vi "Build Installer with API.vi"(8 "error in (no error)":errorcluster, 11 "PostBuildSupport in":refnum<class "PostBuildSupport.lvclass">) -> (0 "error out":errorcluster, 3 "PostBuildSupport out":refnum<class "PostBuildSupport.lvclass">)   [LabVIEW 2019, in "PostBuildSupport.lvclass"]
uses:
  PostBuildSupport.lvclass
  PostBuildSupport.lvclass/PostBuildSupport.ctl
  <vilib>/AppBuilder/IB_Classes/Destination/IB_Destination.lvclass
  <vilib>/AppBuilder/IB_Classes/Source/IB_Source.lvclass
  <vilib>/AppBuilder/IB_Classes/Dest_NI_NIPath/Dest_NI_NIPath.lvclass
  <vilib>/AppBuilder/AB_API/EXE/NI_AB_API_EXE.lvclass
  <vilib>/AppBuilder/IB_Classes/Installer/Installer.lvclass
panel:
  in  "Cancel Button":bool
  out "Progress Bar":u8(slide) caption="The build is complete. You can locate the build at\nC:\\user\\patrick\\git\\PPMS-Monitor-and-Control\\builds\\PPMS Monitor and Control\\Application." scale=0.0..100.0
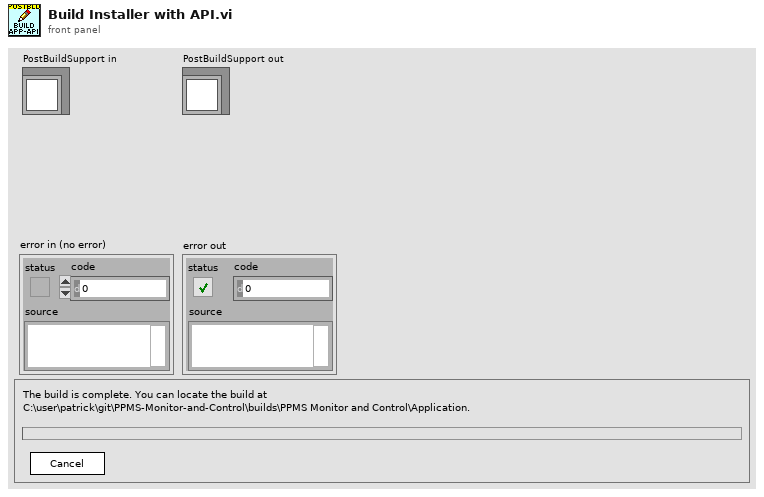
[diagram p1: front panel]
types:
  T1 = enum8{"Enabled", "Disabled", "Disabled and Grayed Out"}
  T2 = typedef "IB_Installer.ctl" = cluster{"Destination":refnum<class "IB_Destination.lvclass">[], "Source":refnum<class "IB_Source.lvclass">[], "buildObject":T3, "defaultDir":string, "platform":string, "author":string, "productName":string, "buildSpecName":string, "hide":bool, "requireLVDevSys":bool, "autoIncrement":bool, "includeError":bool, "readmeID":string, "buildLocation":path, "readmePath":path, "mediaSize":u16, "language":T4, "productVersion":T5, "preview":bool, "programmatic":bool, "progressBarEvents":T6, "userLog_Path":path, "shortcutAddresses":T8[], "EXE_Install Address":string, "EXE_Uninstall Address":string, "additional NIPaths":refnum<class "Dest_NI_NIPath.lvclass">[], "web service itemIDs":string[], "installerName":string}
  T3 = typedef "ItemRef.ctl" = u64
  T4 = typedef "CDK_sTypeDef_Languages.ctl" = u16
  T5 = typedef "CDK_sTypeDef_ProductVersion.ctl" = cluster{"Major":u8, "Minor":u8, "Update":u16}
  T6 = typedef "provcom_ProgressBar_Events.ctl" = cluster{"newJob":refnum<user-event>, "newItem":refnum<user-event>, "errorMsg":T7, "cancel":refnum<user-event>}
  T7 = typedef "mxLvBuildError.ctl" = refnum<user-event>
  T8 = typedef "CDK_sTypeDef_ShortcutAddress.ctl" = cluster{"file":string, "shortcut":string}
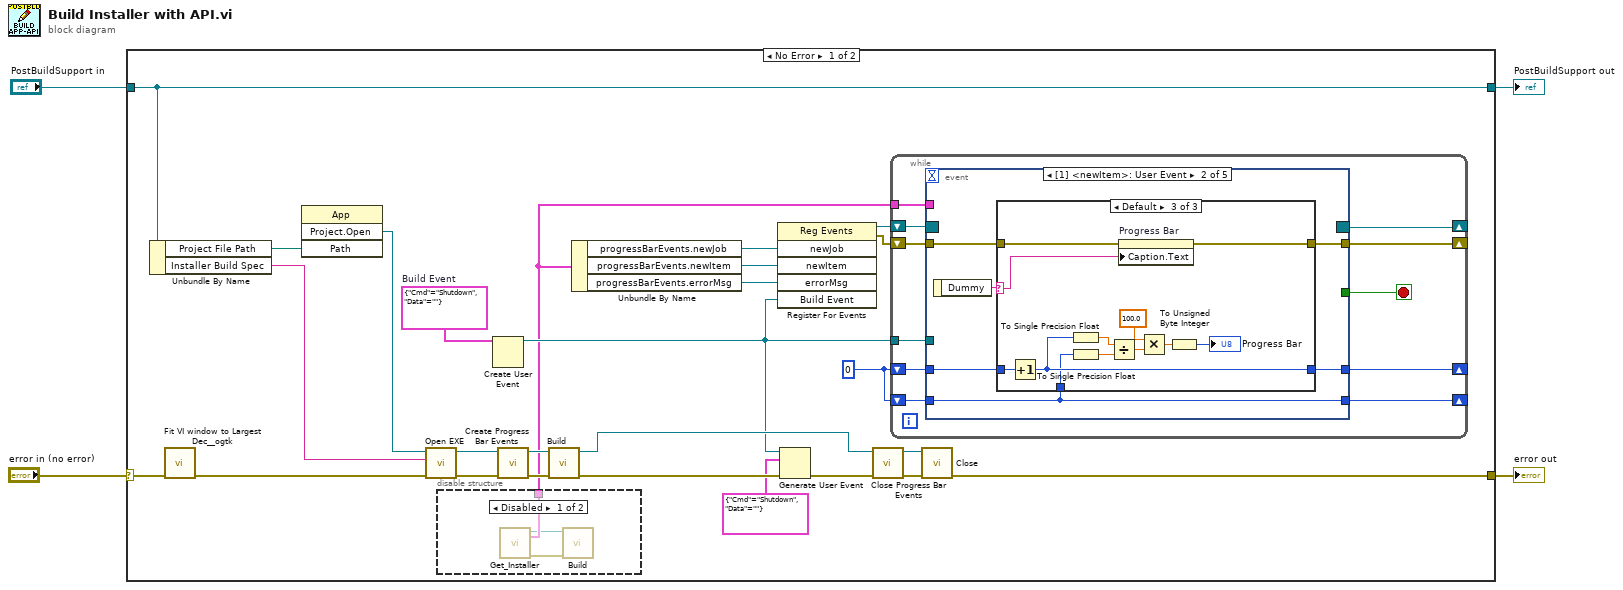
[diagram p0: block diagram]
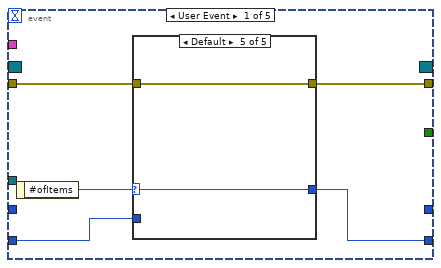
[diagram p3: hidden frame]
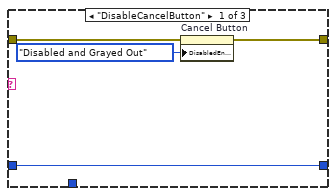
[diagram p8: hidden frame]
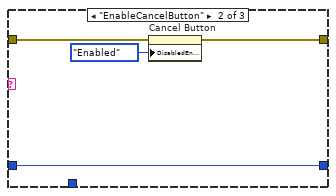
[diagram p9: hidden frame]
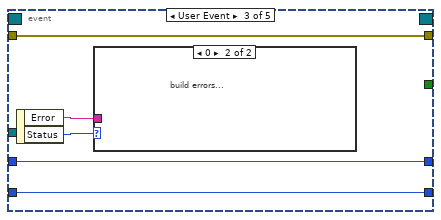
[diagram p10: hidden frame]
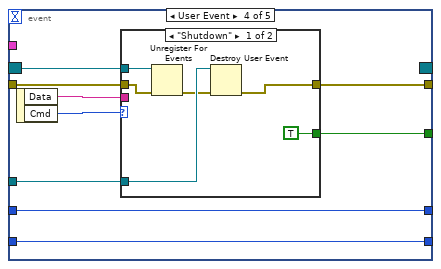
[diagram p12: hidden frame]
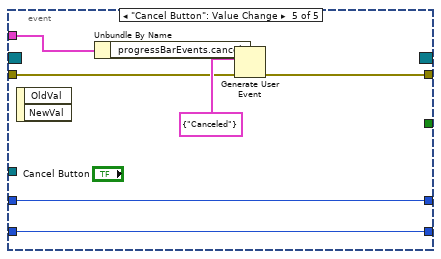
[diagram p14: hidden frame]
diagram:
  n1 = case shown="No Error" "error in (no error)" {
    selector: "error in (no error)" -> [w27 w115]
    tunnel: "PostBuildSupport in" -> [w30 w114]
    tunnel: [w29 w115] -> w2
    tunnel: [w30 w114] -> w1
    frame No Error {
      w15 = cluster{"Cmd":enum16{"Shutdown"}, "Data":string} {"Cmd"=enum."Shutdown", "Data"=""}  # Build Event
      w14 = 0 ("#ofItems")
      n2 = Unbundle By Name(w30) -> ("Project File Path"=w6:path, "Installer Build Spec"=w5:string)
      n3 = call <userlib>:"Fit VI window to Largest Dec__ogtk.vi"("error in (no error)"=w27) -> ("error out"=w26:errorcluster)  [unwired: 5 in, 1 out]
      n4 = invoke class="App" method="Project.Open"("Path"=w6) -> ("Project:Open"=w28:refnum<vi>)  [unwired: 3 in, 3 out]
      n5 = call <vilib>:"Open EXE.vi"("error in (no error)"=w26, "Build specification name"=w5, "Project Refnum"=w28) -> ("error out"=w9:errorcluster, "EXE out"=w7:refnum<class "NI_AB_API_EXE.lvclass">)  [unwired: 7 in]
      n6 = disable-structure shown="Disabled" {
        disable-tunnel: [w33 _] -> w8
        frame Disabled {
          n7 = call <vilib>:"Get_Installer.vi"() -> ("error out"=w32:errorcluster, "data"=w33:T2, "Installer out"=w31:refnum<class "Installer.lvclass">)  [unwired: 9 in]
          n8 = call-dynamic "Build.vi"("error in (no error)"=w32, "Class in"=w31) -> ()  [unwired: 6 in, 4 out]
        }
        frame Enabled {
        }
      }
      n9 = Create User Event(user event datatype=w15) -> (user event=w11:refnum<user-event>)  [unwired: 1 in, 1 out]
      n10 = call-dynamic "Create Progress Bar Events.vi"("error in (no error)"=w9, "NI_AB_API_Build in"=w7) -> ("error out"=w21:errorcluster, "NI_AB_API_Build out"=w25:refnum<class "NI_AB_API_EXE.lvclass">)  [unwired: 7 in, 1 out]
      n11 = call-dynamic "Build.vi"("error in (no error)"=w21, "EXE in"=w25) -> ("error out"=w13:errorcluster, "EXE out"=w24:refnum<class "NI_AB_API_EXE.lvclass">)  [unwired: 6 in, 2 out]
      n12 = Unbundle By Name(w8) -> ("progressBarEvents.newJob"=w20:refnum<user-event>, "progressBarEvents.newItem"=w19:refnum<user-event>, "progressBarEvents.errorMsg"=w18:T7)
      n13 = register-events(w20, w19, w18, w11) -> (reference out=w17:refnum<event-registration>, error out=w16:errorcluster)  [unwired: 2 in]
      n14 = Generate User Event(user event=w11, event data cluster=cluster{"Cmd":enum16{"Shutdown"}, "Data":string} {"Cmd"=enum."Shutdown", "Data"=""} ("event data"), error in=w13) -> (error out=w12:errorcluster)  [unwired: 1 in, 1 out]
      n15 = call-dynamic "Close Progress Bar Events.vi"("error in (no error)"=w12, "NI_AB_API_Build in"=w24) -> ("error out"=w22:errorcluster, "NI_AB_API_Build out"=w23:refnum<class "NI_AB_API_EXE.lvclass">)  [unwired: 8 in]
      n16 = while {
        shift-right: [w44] -> _
        shift-left: w16 -> [w41]
        shift-right: [w43] -> _
        shift-left: w17 -> [w42]
        shift-right: [w39] -> _
        shift-left: w14 -> [w36]
        shift-right: [w38] -> _
        shift-left: w14 -> [w37]
        tunnel: w11 -> [w35]
        tunnel: w8 -> [w34]
        stop <- w40 stop-if-true
        n17 = event shown="[1] <newItem>: User Event" {
          selector: w42 -> [_ _ _ w95 _]
          dyn-events: [_ _ _ _ _] -> w43
          timeout: _ -> [_ _ _ _ _]
          tunnel: [w48 w61 w90 w94 w111] -> w44
          tunnel: w41 -> [w49 w60 w90 w93 w107]
          tunnel: [_ _ _ w97 _] -> w40
          tunnel: [w46 w63 w88 w98 w110] -> w39
          tunnel: [_ w64 w89 w99 w109] -> w38
          tunnel: w37 -> [_ w62 w89 w99 w109]
          tunnel: w36 -> [w45 w63 w88 w98 w110]
          tunnel: w35 -> [_ _ _ w91 _]
          tunnel: w34 -> [_ _ _ _ w108]
          event User Event {
            n18 = event-data() -> ("#ofItems"=w47:i32)  [unwired: 1 in]
            n19 = case shown="Default" w47 {
              selector: w47 -> [w51 w53 w55 _ w59]
              tunnel: w49 -> [w50 w52 w54 w57 w58]
              tunnel: [w50 w52 w54 w57 w58] -> w48
              tunnel: [w51 w53 w55 w56 w59] -> w46
              tunnel: w45 -> [_ _ _ w56 _]
              frame -1 {
                # "Canceled response"
              }
              frame -2 {
              }
              frame -3 {
              }
              frame -4 {
              }
              frame Default {
              }
            }
          }
          event User Event {
            n20 = event-data() -> ("Dummy"=w65:string)  [unwired: 1 in]
            n21 = case shown="Default" w65 {
              selector: w65 -> [_ _ w76]
              tunnel: w62 -> [w68 w72 w83]
              tunnel: [w68 w72 w82] -> w64
              tunnel: w63 -> [_ _ w81]
              tunnel: [w66 w70 w74] -> w61
              tunnel: w60 -> [w67 w71 w75]
              frame "DisableCancelButton" {
                n22 = property on="Cancel Button" class="Bool"(error in=w67, "DisabledEnum"=T1."Disabled and Grayed Out" ("Disabled")) -> (error out=w66:errorcluster)  [unwired: 1 in, 1 out]
              }
              frame "EnableCancelButton" {
                n23 = property on="Cancel Button" class="Bool"(error in=w71, "DisabledEnum"=T1."Enabled" ("Disabled")) -> (error out=w70:errorcluster)  [unwired: 1 in, 1 out]
              }
              frame Default {
                n24 = Increment(x=w83) -> (x+1=w82:i32)
                n25 = To Single Precision Float(number=w82) -> (single precision float=w79:sgl)
                n26 = To Single Precision Float(number=w81) -> (single precision float=w78:sgl)
                n27 = Divide(x=w79, y=w78) -> (x/y=w80:sgl)
                n28 = property on="Progress Bar" class="Slide (strict)"(error in=w75, "Caption.Text"=w76) -> (error out=w74:errorcluster)  [unwired: 1 in, 1 out]
                n29 = Multiply(x=sgl 100.0, y=w80) -> (x*y=w85:sgl)
                n30 = To Unsigned Byte Integer(number=w85) -> (unsigned 8bit integer=→"Progress Bar":u8)
              }
            }
          }
          event User Event {
            n31 = event-data() -> ("Error"=w86:string, "Status"=w87:i32)  [unwired: 1 in]
            n32 = case shown="0" w87 {
              tunnel: w86 -> [_ _]
              frame Default {
              }
              frame 0 {
                # "build errors..."
              }
            }
          }
          event User Event {
            n33 = event-data() -> ("Data"=w92:string, "Cmd"=w96:enum16{"Shutdown"})  [unwired: 1 in]
            n34 = case shown="\"Shutdown\"" w96 {
              tunnel: [TRUE _] -> w97
              tunnel: w95 -> [w104 _]
              tunnel: [w100 w106] -> w94
              tunnel: w93 -> [w103 w106]
              tunnel: w92 -> [_ _]
              tunnel: w91 -> [w102 _]
              frame "Shutdown" {
                n35 = Unregister For Events(event registration refnum=w104, error in=w103) -> (error out=w101:errorcluster)
                n36 = Destroy User Event(user event=w102, error in=w101) -> (error out=w100:errorcluster)
              }
              frame Default {
              }
            }
          }
          event "Cancel Button": Value Change {
            n37 = event-data() -> ()  [unwired: 1 in, 2 out]
            n38 = Unbundle By Name(w108) -> ("progressBarEvents.cancel"=w112:refnum<user-event>)
            n39 = Generate User Event(user event=w112, event data cluster=cluster{"Dummy":string} {"Dummy"="Canceled"} ("event data"), error in=w107) -> (error out=w111:errorcluster)  [unwired: 1 in, 1 out]
          }
        }
      }
      n40 = call-dynamic "Close.vi"("error in (no error)"=w22, "EXE in"=w23) -> ("error out"=w29:errorcluster)  [unwired: 9 in]
    }
    frame Error {
    }
  }
  "error out" <- w2
  "PostBuildSupport out" <- w1
